vi "Get newest data.vi"(4 "target path":path, 5 "End time":string, 6 "source path":path, 7 "Start time":string, 10 "Previous info":T2={"Last time in range?"=FALSE, "Date"="", "Start index"=1757}, 11 "all rows":string[][](array[string])) -> (2 "New Info":T1, 3 "newest rows":string[][](array[string]))   [LabVIEW 2014]
uses:
  TypeDefs/Data Info.ctl
  <vilib>/Utility/file.llb/Write To Spreadsheet File (string).vi
panel:
  out "concatenated string":string
  out "write path":path
  out "string":string
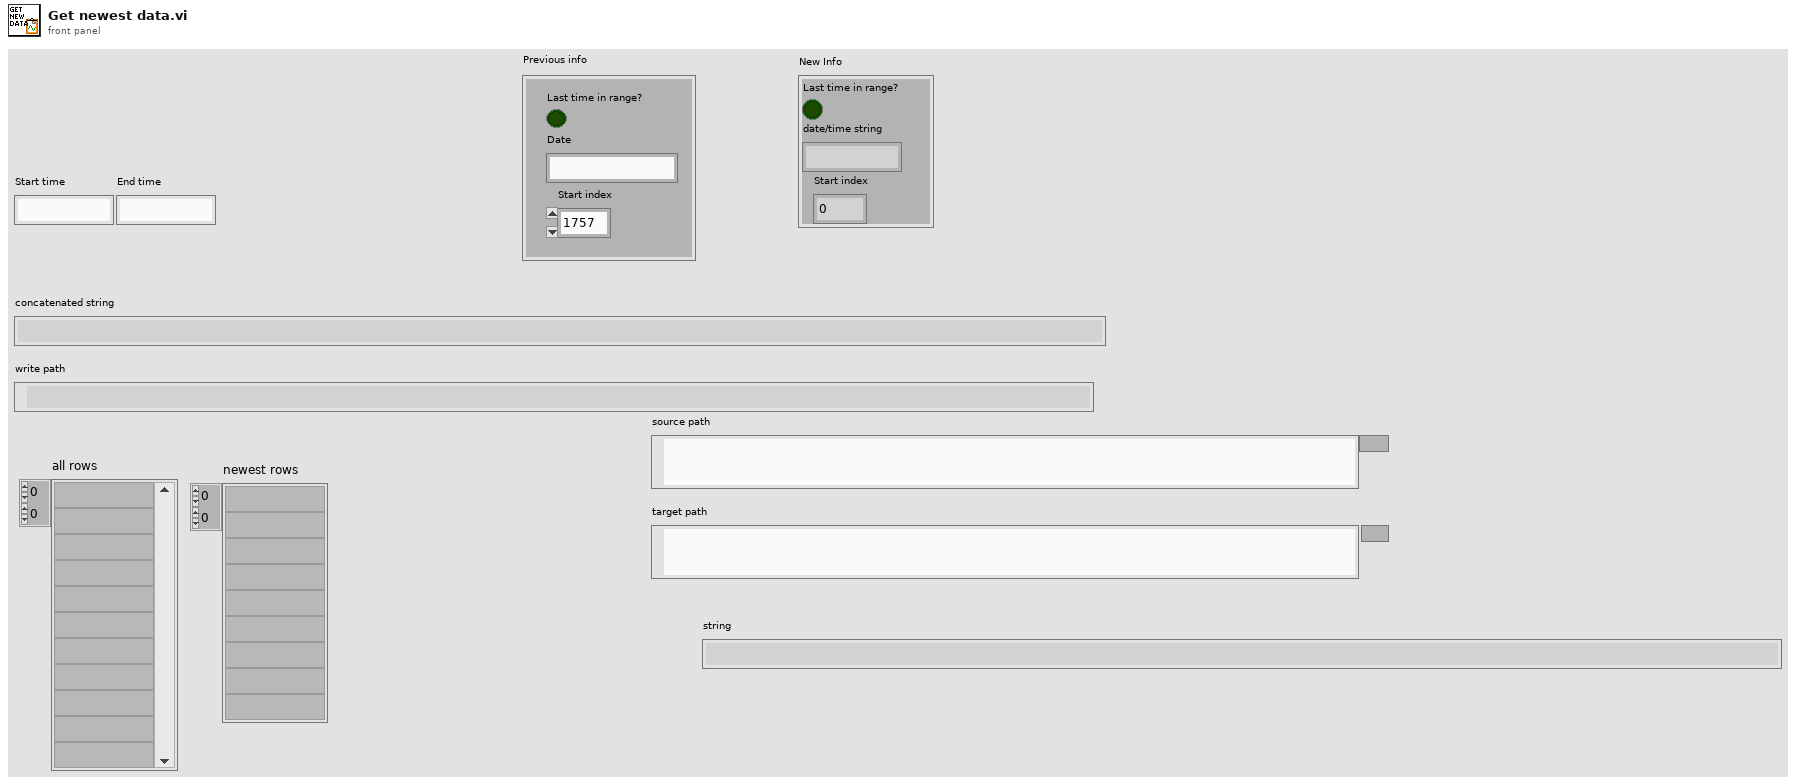
[diagram p1: front panel]
types:
  T1 = cluster{"Last time in range?":bool, "date/time string":string, "Start index":i32}
  T2 = typedef "Data Info.ctl" = cluster{"Last time in range?":bool, "Date":string, "Start index":i32}
  T3 = typedef "LVDateTimeRec.ctl" = cluster{"fractional second":dbl, "second":i32, "minute":i32, "hour":i32, "day of month":i32, "month":i32, "year":i32, "day of week":i32, "day of year":i32, "DST":i32}
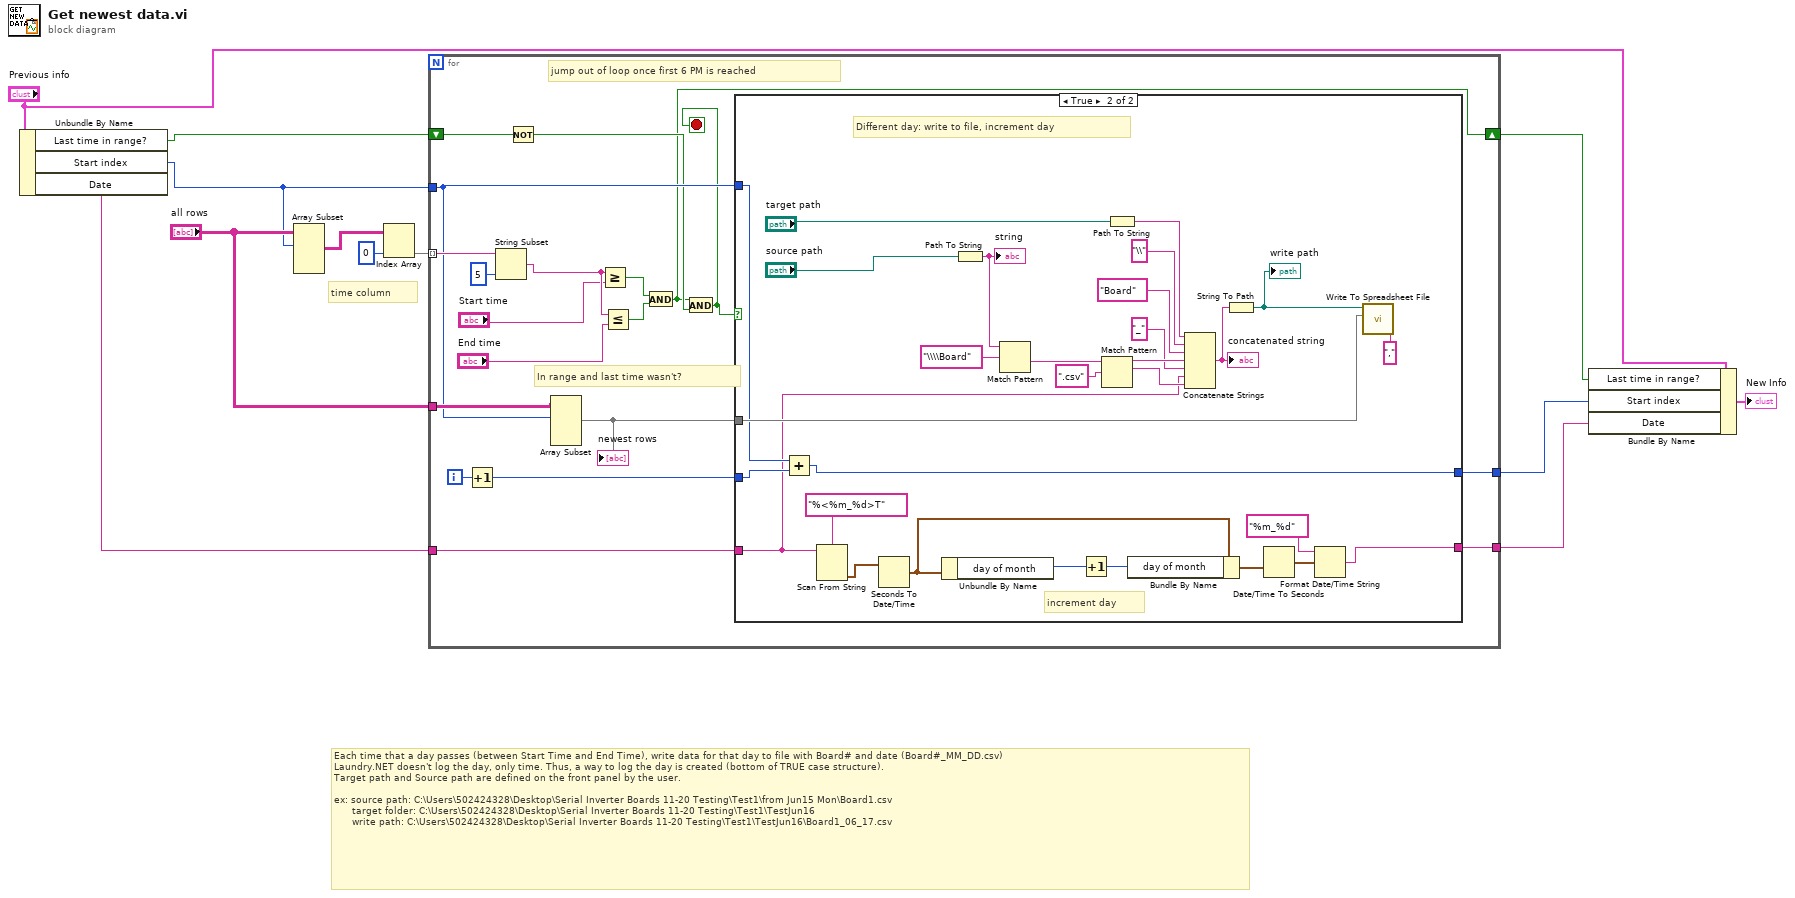
[diagram p0: block diagram]
diagram:
  # "time column"
  # "Each time that a day passes (between Start Time and End Time), write data for that day to file with Board# and date (Board#_MM_DD.csv)\nLaundry.NET doesn't log the day, only time. Thus, a way to log the day is created (bottom of TRUE case structure).\nTarget path and Source path are defined on the front panel by the user.\n\nex: source path: C:\\Users\\502424328\\Desktop\\Serial Inverter Boards 11-20 Testing\\Test1\\from Jun15 Mon\\Board1.csv \n      target folder: C:\\Users\\502424328\\Desktop\\Serial Inverter Boards 11-20 Testing\\Test1\\TestJun16\n      write path: C:\\Users\\502424328\\Desktop\\Serial Inverter Boards 11-20 Testing\\Test1\\TestJun16\\Board1_06_17.csv"
  n1 = Unbundle By Name("Previous info") -> ("Last time in range?"=w8:bool, "Start index"=w7:i32, "Date"=w6:string)
  n2 = Array Subset(array="all rows", index (row)=w7) -> (w10:string[][])  [unwired: 3 in]
  n3 = Index Array(array=w10, index (col)=0 ("disabled index (col)")) -> (element=w12:string[])  [unwired: 1 in]
  n4 = for {
    tunnel: w12 -> [w28] mode=indexing
    tunnel: [w27] -> w3
    tunnel: "all rows" -> [w26]
    tunnel: w7 -> [w20]
    tunnel: w6 -> [w18]
    tunnel: [w17] -> w2
    shift-right: [w13] -> w4
    shift-left: w8 -> [w16]
    i -> [w24]
    stop <- w14 stop-if-true
    # "In range and last time wasn't?"
    # "jump out of loop once first 6 PM is reached"
    n5 = Increment(x=w24) -> (x+1=w19:i32)
    n6 = String Subset(string=w28, length (rest)=5 ("length (rest)")) -> (substring=w23:string)  [unwired: 1 in]
    n7 = Not(x=w16) -> (.not. x?=w15:bool)
    n8 = Array Subset(array=w26, index (row)=w20) -> (w25:string[][])  [unwired: 3 in]
    "newest rows" <- w25
    n9 = Greater Or Equal?(x=w23, y="Start time") -> (x >= y?=w30:bool)
    n10 = Less Or Equal?(x=w23, y="End time") -> (x <= y?=w29:bool)
    n11 = And(x=w30, y=w29) -> (x .and. y?=w13:bool)
    n12 = And(x=w13, y=w15) -> (x .and. y?=w14:bool)
    n13 = case shown="True" w14 {
      tunnel: [w33 w45] -> w27
      tunnel: w25 -> [_ w48]
      tunnel: w20 -> [w33 w47]
      tunnel: w19 -> [_ w46]
      tunnel: w18 -> [w32 w35]
      tunnel: [w32 w36] -> w17
      frame False {
        # "Same day, don't write to file"
      }
      frame True {
        # "increment day"
        # "Different day: write to file, increment day"
        n14 = Add(x=w47, y=w46) -> (x+y=w45:i32)
        n15 = Scan From String(format string="%<%m_%d>T", input string=w35) -> (output 1=w43:timestamp)  [unwired: 3 in, 3 out]
        n16 = Seconds To Date/Time(time stamp (now)=w43) -> (date time rec=w41:T3)  [unwired: 1 in]
        n17 = Unbundle By Name(w41) -> ("day of month"=w42:i32)
        n18 = Path To String(path="source path") -> (string=w51:string)
        "string" <- w51
        n19 = Match Pattern(string=w51, regular expression="\\\\Board") -> (after substring=w59:string)  [unwired: 1 in, 3 out]
        n20 = Increment(x=w42) -> (x+1=w40:i32)
        n21 = Match Pattern(string=w59, regular expression=".csv") -> (before substring=w57:string, match substring=w55:string)  [unwired: 1 in, 2 out]
        n22 = Path To String(path="target path") -> (string=w60:string)
        n23 = Bundle By Name(cluster=w41, "day of month"=w40) -> (w39:T3)
        n24 = Concatenate Strings(w60, "\\" ("string"), "Board" ("string"), w57, "_" ("string"), w35, w55) -> (w61:string)
        "concatenated string" <- w61
        n25 = String To Path(string=w61) -> (path=w62:path)
        "write path" <- w62
        n26 = Date/Time To Seconds(2:w39) -> (0:w38:timestamp)  [unwired: 1 in]
        n27 = Format Date/Time String(time format string (%c)="%m_%d", seconds (now)=w38) -> (date/time string=w36:string)  [unwired: 1 in]
        n28 = call-poly <vilib>:"Write To Spreadsheet File.vi"("delimiter (\\t)"="," ("delimiter (\\t)"), "2D data"=w48, "file path (dialog if empty)"=w62) -> ()  [unwired: 5 in, 1 out]
      }
    }
  }
  n29 = Bundle By Name(cluster="Previous info", "Last time in range?"=w4, "Start index"=w3, "Date"=w2) -> (→"New Info":T2)
